vi "base.vi"() -> ()   [LabVIEW 2021]
uses:
  <vilib>/Utility/file.llb/Write Delimited Spreadsheet (I64).vi
panel:
  out "Array":i32[][](array[numeric])
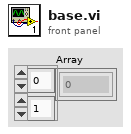
[diagram p1: front panel]
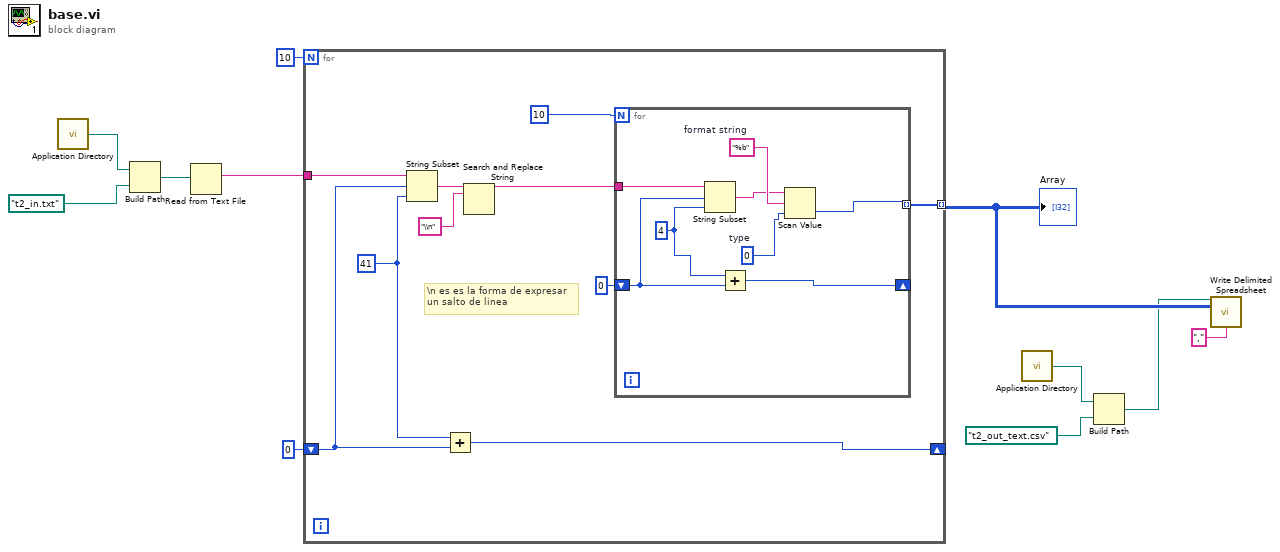
[diagram p0: block diagram]
diagram:
  n1 = call <vilib>:"Application Directory.vi"() -> ("Application Directory"=w10:path)
  n2 = Build Path(base path=w10, name or relative path=path "t2_in.txt" ("file (use dialog)")) -> (appended path=w8:path)
  n3 = Read from Text File(file (use dialog)=w8) -> (text=w11:string)  [unwired: 3 in, 3 out]
  n4 = for {
    N: 10 -> [_]
    tunnel: w11 -> [w21]
    shift-right: [w19] -> _
    shift-left: 0 -> [w18]
    tunnel: [w12] -> w5 mode=indexing
    w20 = 41 ("length (rest)")
    # "\\n es es la forma de expresar\nun salto de linea"
    n5 = String Subset(string=w21, offset (0)=w18, length (rest)=w20) -> (substring=w15:string)
    n6 = Add(x=w20, y=w18) -> (x+y=w19:i32)
    n7 = Search and Replace String(input string=w15, search string="\\n" ("substring (\"\")")) -> (result string=w13:string)  [unwired: 6 in, 3 out]
    n8 = for {
      N: 10 -> [_]
      tunnel: w13 -> [w29]
      shift-right: [w24] -> _
      shift-left: 0 ("length (rest)") -> [w23]
      tunnel: [w22] -> w12 mode=indexing
      w27 = 0  # type
      w28 = "%b"  # format string
      w25 = 4 ("length (rest)")
      n9 = String Subset(string=w29, offset (0)=w23, length (rest)=w25) -> (substring=w26:string)
      n10 = Add(x=w25, y=w23) -> (x+y=w24:i32)
      n11 = Scan Value(string=w26, format string=w28, default (0 dbl)=w27) -> (value=w22:i32)  [unwired: 1 out]
    }
  }
  "Array" <- w5
  n12 = call <vilib>:"Application Directory.vi"() -> ("Application Directory"=w4:path)
  n13 = Build Path(base path=w4, name or relative path=path "t2_out_text.csv" ("file (use dialog)")) -> (appended path=w2:path)
  n14 = call-poly <vilib>:"Write Delimited Spreadsheet.vi"("file path (dialog if empty)"=w2, "2D data"=w5, "delimiter (\\t)"="," ("delimiter (\\t)")) -> ()  [unwired: 11 in, 2 out]
